vi "PowerShell dotNET.vi"() -> ()   [LabVIEW 2018]
uses:
  System.Management.Automation
panel:
  out "error out":errorcluster
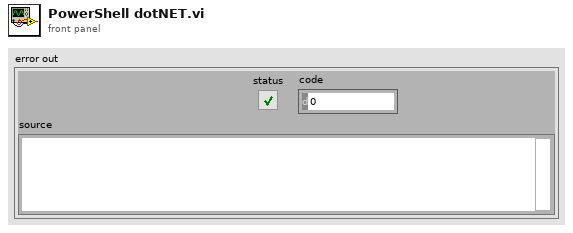
[diagram p1: front panel]
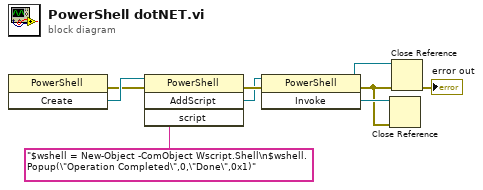
[diagram p0: block diagram]
diagram:
  n1 = invoke class="PowerShell" method="Create"() -> (error out=w6:errorcluster, "Create"=w9:refnum<k24>)  [unwired: 3 in, 1 out]
  n2 = invoke class="PowerShell" method="AddScript"(reference=w9, error in=w6, "script"="$wshell = New-Object -ComObject Wscript.Shell\n$wshell.Popup(\"Operation Completed\",0,\"Done\",0x1)") -> (error out=w5:errorcluster, "AddScript"=w3:refnum<k24>)  [unwired: 1 in, 2 out]
  n3 = invoke class="PowerShell" method="Invoke"(reference=w3, error in=w5) -> (reference out=w7:refnum<k24>, error out=w2:errorcluster, "Invoke"=w8:refnum<k24>)  [unwired: 1 in]
  n4 = Close Reference(reference=w8, error in (no error)=w2) -> ()  [unwired: 1 out]
  n5 = Close Reference(reference=w7, error in (no error)=w2) -> (error out=→"error out":errorcluster)
